vi "Accelerator Shutter Open_Close.vi"(8 "error in (no error)":errorcluster, 10 "ON/OFF":bool=TRUE, 11 "Control-Client in":refnum<class "Control-Client.lvclass">) -> (0 "error out":errorcluster, 3 "Control-Client out":refnum<class "Control-Client.lvclass">)   [LabVIEW 2015, in "Control-Client.lvclass"]
uses:
  Control-Client.lvclass
  dependecies/ControlsVIs/Clusters-def/Message types.ctl
  dependecies/ControlsVIs/Clusters-def/SERVER-Commands.ctl
  Control-Server/Control-Server.lvclass
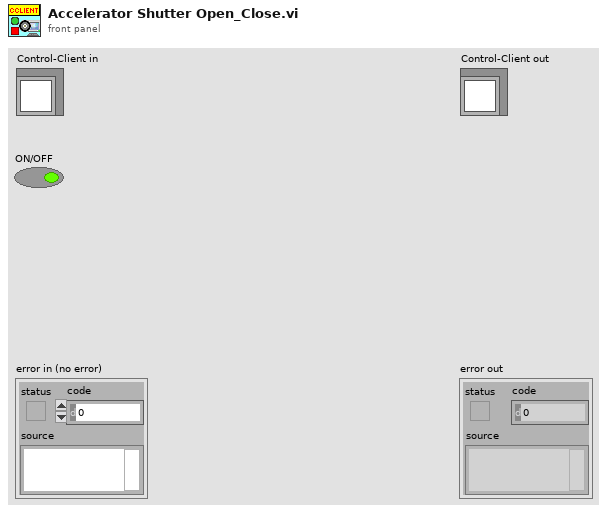
[diagram p1: front panel]
types:
  T1 = typedef "Control-Server.lvclass/SERVER-Commands.ctl" = string
  T2 = typedef "Message types.ctl" = string
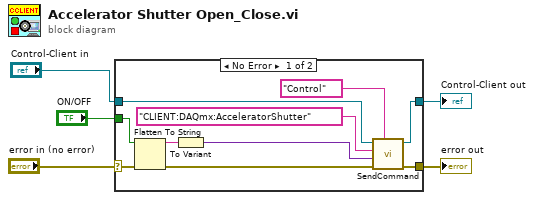
[diagram p0: block diagram]
diagram:
  n1 = case shown="No Error" "error in (no error)" {
    selector: "error in (no error)" -> [w8 w17]
    tunnel: [w14 w17] -> w4
    tunnel: [w13 w16] -> w2
    tunnel: "Control-Client in" -> [w15 w16]
    tunnel: "ON/OFF" -> [w9 _]
    frame No Error {
      n2 = Flatten To String(anything=w9, error in (no error)=w8) -> (data string=w6:string, error out=w7:errorcluster)  [unwired: 2 in, 1 out]
      n3 = To Variant(anything=w6) -> (Variant=w12:variant)
      n4 = call "SendCommand.vi"("Message type"=T2 "Control", "error in (no error)"=w7, "data"=w12, "Command"=T1 "CLIENT:DAQmx:AcceleratorShutter" ("Commands"), "Control-Client in"=w15) -> ("error out"=w14:errorcluster, "Control-Client out"=w13:refnum<class "Control-Client.lvclass">)  [unwired: 5 in]
    }
    frame Error {
    }
  }
  "error out" <- w4
  "Control-Client out" <- w2
